vi "Create Q Reference (SubVI).vi"() -> (3 "Image Queue":T1)   [LabVIEW 2020]
uses:
  Controls (HOST)/Image Queue Bundle.ctl
  Controls (HOST)/Data to Disk Bundle.ctl
  Controls (HOST)/File Name Prefix.ctl
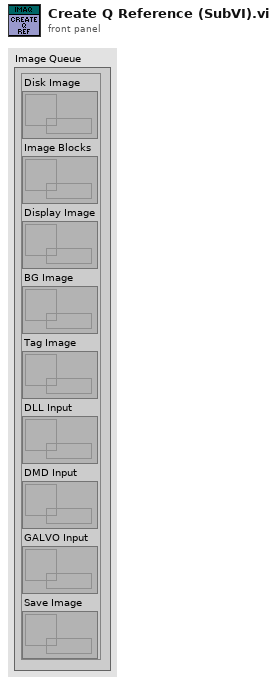
[diagram p1: front panel]
types:
  T1 = typedef "Image Queue Bundle.ctl" = cluster{"Disk Image":refnum<queue>, "Image Blocks":refnum<queue>, "Display Image":refnum<queue>, "BG Image":refnum<queue>, "Tag Image":refnum<queue>, "DLL Input":refnum<queue>, "DMD Input":refnum<queue>, "GALVO Input":refnum<queue>, "Save Image":refnum<queue>}
  T2 = typedef "Data to Disk Bundle.ctl" = cluster{"Frame Number":u64, "Time Stamp (us)":u64, "Image Data":u64[], "Contour":u32[], "Raw Image REF":refnum<data-value>, "Block Image REF":refnum<data-value>, "Block Box":u64[], "SPINE":u32[], "HT Angle":u64[], "Block Position":u64[], "SPINE Count":u32[], "Contour Count":u32[], "SPINE DIR":u8[]}
  T3 = typedef "File Name Prefix.ctl" = cluster{"DateTimeStamp":string, "Genotype 1":string, "Genotype 2":string, "Rig Name":string, "STIM Mode":string, "Light Intensity (%)":i32, "Pixel Resolution (um/pixel)":dbl, "Gamma":dbl, "Yoked File Name":string, "Yoked File Enable":bool, "Output Folder Name":path, "Frame Number":u64, "Time Stamp (us)":u64, "Exp STOP":i32, "Contour":cluster{"X":i32[], "Y":i32[]}[], "SPINE":cluster{"X":dbl[], "Y":dbl[]}[], "Larvae ID":u32[], "Larvae Valid?":bool[], "Image Height":i32, "Image Width":i32, "Pixel Intensity Low":i32, "Pixel Intensity High":i32, "Box Side Low":i32, "Box Side High":i32, "Box W+L Low":i32, "Box W+L High":i32, "Area Low":i32, "Area High":i32, "N SPINE":i32, "BG SUB TH":i32, "Min Contour Points":i32, "STIM Array":dbl[], "Stimulus Label Array":u8[], "Flip Laravae ID":i32[], "IR Intensity":i32}
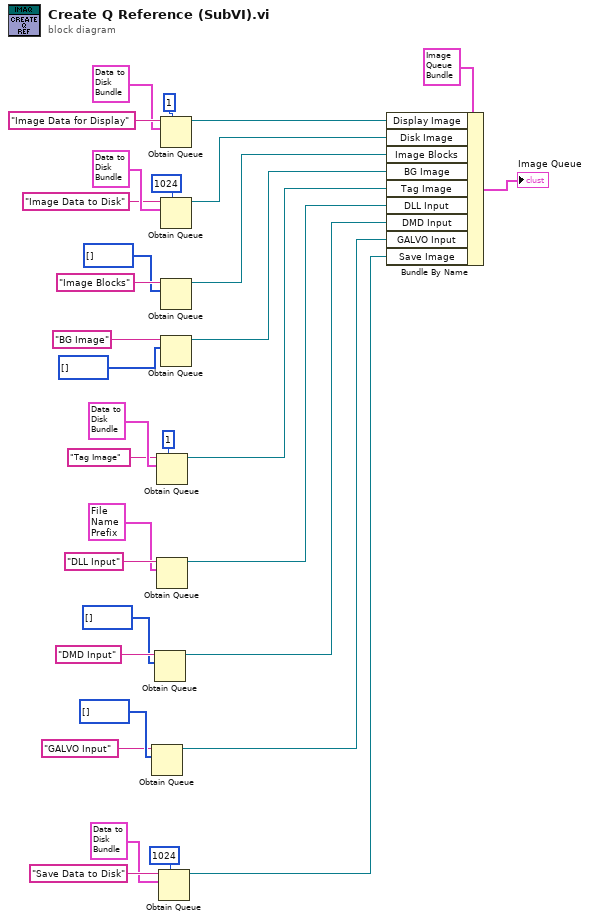
[diagram p0: block diagram]
diagram:
  n1 = Obtain Queue(name (unnamed)="GALVO Input", element data type=i32[] [] ("dmdData")) -> (queue out=w5:refnum<queue>)  [unwired: 3 in, 2 out]
  n2 = Obtain Queue(name (unnamed)="DMD Input", element data type=i32[] [] ("dmdData")) -> (queue out=w8:refnum<queue>)  [unwired: 3 in, 2 out]
  n3 = Obtain Queue(max queue size (-1, unlimited)=1, name (unnamed)="Tag Image", element data type=T2 {"Frame Number"=0, "Time Stamp (us)"=0, "Image Data"=[], "Contour"=[], "Raw Image REF"=refnum, "Block Image REF"=refnum, "Block Box"=[], "SPINE"=[], "HT Angle"=[], "Block Position"=[], "SPINE Count"=[], "Contour Count"=[], "SPINE DIR"=[]} ("Data to Disk")) -> (queue out=w14:refnum<queue>)  [unwired: 2 in, 2 out]
  n4 = Obtain Queue(name (unnamed)="DLL Input", element data type=T3 {"DateTimeStamp"="DateTimeStamp", "Genotype 1"="genotype1", "Genotype 2"="genotype2", "Rig Name"="t21", "STIM Mode"="stimulationMode", "Light Intensity (%)"=100, "Pixel Resolution (um/pixel)"=100.0, "Gamma"=0.2, "Yoked File Name"="none", "Yoked File Enable"=FALSE, "Output Folder Name"=path "", "Frame Number"=0, "Time Stamp (us)"=0, "Exp STOP"=0, "Contour"=[], "SPINE"=[], "Larvae ID"=[], "Larvae Valid?"=[], "Image Height"=0, "Image Width"=0, "Pixel Intensity Low"=0, "Pixel Intensity High"=0, "Box Side Low"=0, "Box Side High"=0, "Box W+L Low"=0, "Box W+L High"=0, "Area Low"=0, "Area High"=0, "N SPINE"=0, "BG SUB TH"=0, "Min Contour Points"=0, "STIM Array"=[], "Stimulus Label Array"=[], "Flip Laravae ID"=[], "IR Intensity"=0} ("DLL Input Param")) -> (queue out=w11:refnum<queue>)  [unwired: 3 in, 2 out]
  n5 = Obtain Queue(max queue size (-1, unlimited)=1024, name (unnamed)="Save Data to Disk", element data type=T2 {"Frame Number"=0, "Time Stamp (us)"=0, "Image Data"=[], "Contour"=[], "Raw Image REF"=refnum, "Block Image REF"=refnum, "Block Box"=[], "SPINE"=[], "HT Angle"=[], "Block Position"=[], "SPINE Count"=[], "Contour Count"=[], "SPINE DIR"=[]} ("Data to Disk")) -> (queue out=w2:refnum<queue>)  [unwired: 2 in, 2 out]
  n6 = Obtain Queue(max queue size (-1, unlimited)=1, name (unnamed)="Image Data for Display", element data type=T2 {"Frame Number"=0, "Time Stamp (us)"=0, "Image Data"=[], "Contour"=[], "Raw Image REF"=refnum, "Block Image REF"=refnum, "Block Box"=[], "SPINE"=[], "HT Angle"=[], "Block Position"=[], "SPINE Count"=[], "Contour Count"=[], "SPINE DIR"=[]} ("Data to Disk")) -> (queue out=w25:refnum<queue>)  [unwired: 2 in, 2 out]
  n7 = Obtain Queue(max queue size (-1, unlimited)=1024, name (unnamed)="Image Data to Disk", element data type=T2 {"Frame Number"=0, "Time Stamp (us)"=0, "Image Data"=[], "Contour"=[], "Raw Image REF"=refnum, "Block Image REF"=refnum, "Block Box"=[], "SPINE"=[], "HT Angle"=[], "Block Position"=[], "SPINE Count"=[], "Contour Count"=[], "SPINE DIR"=[]} ("Data to Disk")) -> (queue out=w26:refnum<queue>)  [unwired: 2 in, 2 out]
  n8 = Obtain Queue(name (unnamed)="Image Blocks", element data type=u8[] []) -> (queue out=w22:refnum<queue>)  [unwired: 3 in, 2 out]
  n9 = Obtain Queue(name (unnamed)="BG Image", element data type=u64[] [] ("data value")) -> (queue out=w18:refnum<queue>)  [unwired: 3 in, 2 out]
  n10 = Bundle By Name(cluster=T1 {"Disk Image"=refnum, "Image Blocks"=refnum, "Display Image"=refnum, "BG Image"=refnum, "Tag Image"=refnum, "DLL Input"=refnum, "DMD Input"=refnum, "GALVO Input"=refnum, "Save Image"=refnum}, "Display Image"=w25, "Disk Image"=w26, "Image Blocks"=w22, "BG Image"=w18, "Tag Image"=w14, "DLL Input"=w11, "DMD Input"=w8, "GALVO Input"=w5, "Save Image"=w2) -> (→"Image Queue":T1)
